vi "XY Fitting.vi"() -> ()   [LabVIEW 2020]
uses:
  <vilib>/Utility/miscctls.llb/LVAnnotationListTypeDef.ctl
  global/SettingVariable.vi
  <vilib>/Analysis/NI_AALPro.lvlib
panel:
  out "历史波形图":cluster{dbl, dbl, dbl[][]}(graph)
  out "左选标时刻":timestamp caption="左选标时刻：" format="%<%.2X %x>T"
  out "数据点数":i32 caption="数据点数："
  out "残差":dbl caption="残差："
  out "斜率":dbl caption="斜率："
  in  "在线数据":bool
  out "采样间隔":dbl
  out "开始时间":timestamp
  in  "x轴选择":u16(ring) caption="x轴选择："
  in  "y轴选择":u16(ring) caption="y轴选择："
  in  "打开文件":bool
  out "XY 图":cluster{dbl[], "Best Linear Fit":dbl[]}[](graph)
  out "提示信息":string="打开文件后，拖动波形图中的游标选取显示在XY图上的数据段，通过下拉框选择x和y轴对应的数据。"
  out "文件信息":string
  # "坐标轴与图例"
  # "拟合结果"
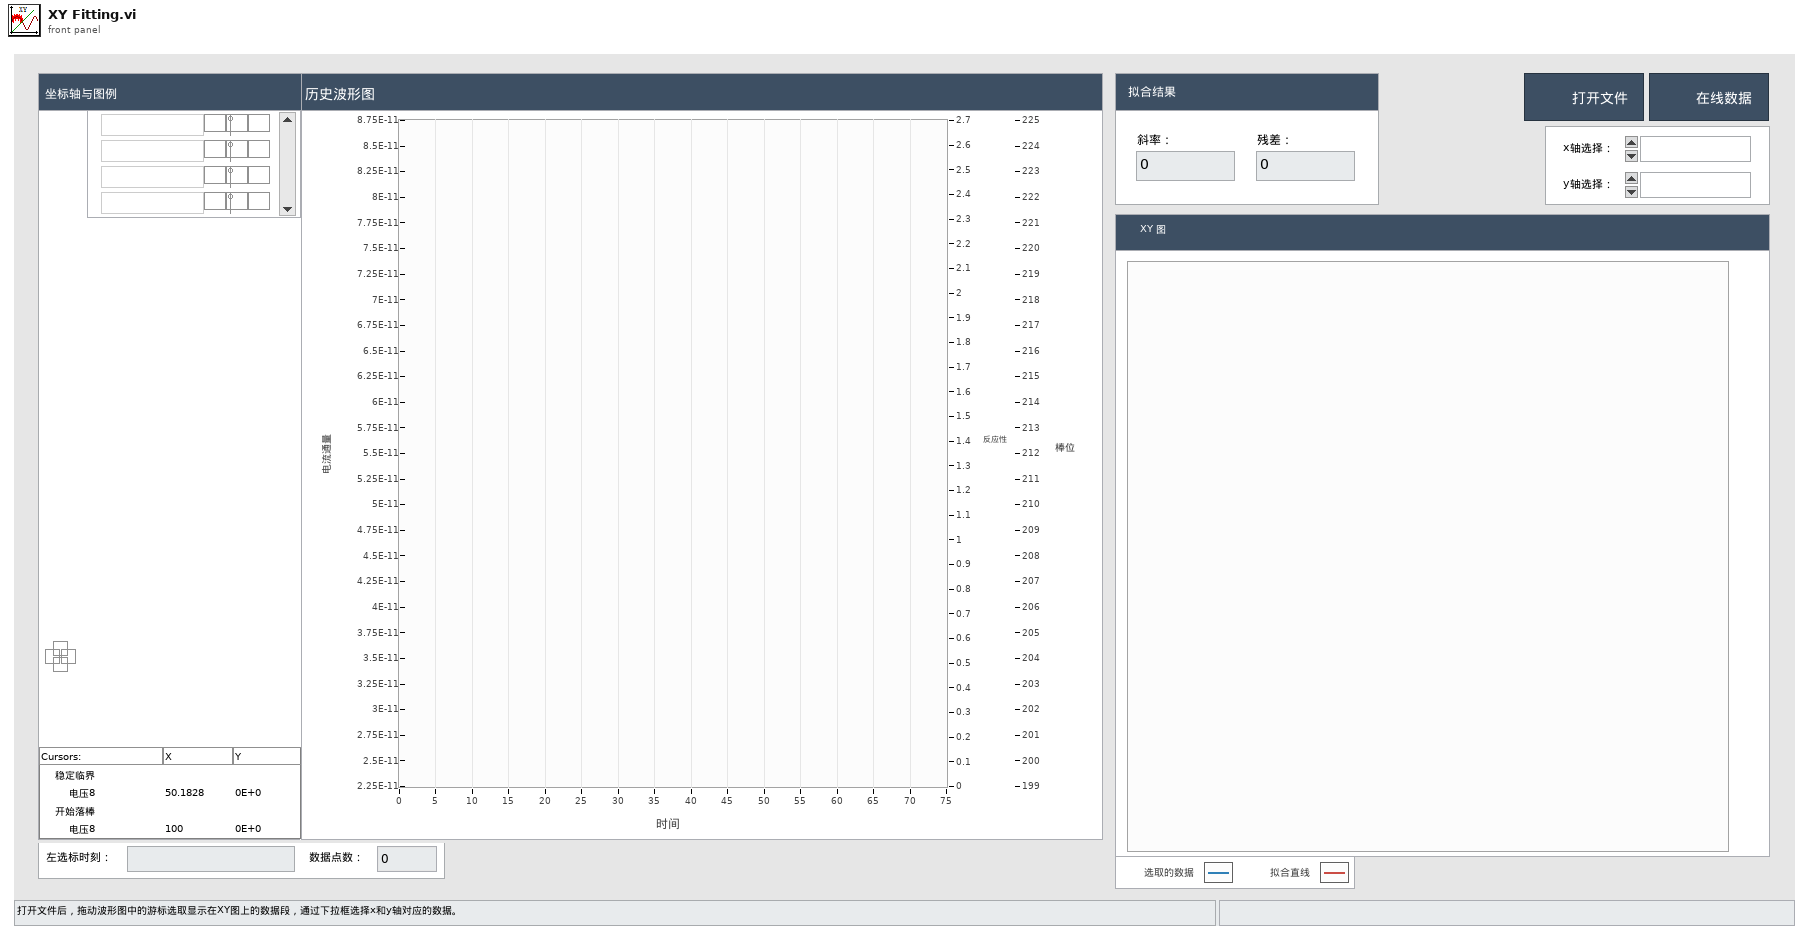
[diagram p1: front panel]
types:
  T1 = typedef "LVAnnotationListTypeDef.ctl" = cluster{"Name":string, "Color":u32, "Style":u8, "Point Style":u8, "Name Visible":bool, "Allow Drag":bool, "Annotation Mode":u32, "Plot":i32, "Index":i32, "Position":cluster{"X":dbl, "Y":dbl}, "X Scale":u32, "Y Scale":u32, "Show Arrow":bool, "Lock Name":bool, "Plot Area":i32, "Label Offset":cluster{"X":dbl, "Y":dbl}}[]
  T2 = cluster{"Name":string, "Color":u32, "Style":u8, "Point Style":u8, "Name Visible":bool, "Allow Drag":bool, "Annotation Mode":u32, "Plot":i32, "Index":i32, "Position":cluster{"X":dbl, "Y":dbl}, "X Scale":u32, "Y Scale":u32, "Show Arrow":bool, "Lock Name":bool, "Plot Area":i32, "Label Offset":cluster{"X":dbl, "Y":dbl}}
  T3 = typedef "LVCursorListTypeDef.ctl" = cluster{"Name":string, "Color":u32, "Style":u8, "Point Style":u8, "Name Visible":bool, "Allow Drag":bool, "Cursor Mode":u32, "Plot":i32, "Index":i32, "Position":cluster{"X":dbl, "Y":dbl}, "X Scale":u32, "Y Scale":u32, "Watch Plots":i32[], "Watch All Plots":bool, "Plot Area":i32, "Label Offset":cluster{"X":dbl, "Y":dbl}}[]
  T4 = cluster{"Name":string, "Color":u32, "Style":u8, "Point Style":u8, "Name Visible":bool, "Allow Drag":bool, "Cursor Mode":u32, "Plot":i32, "Index":i32, "Position":cluster{"X":dbl, "Y":dbl}, "X Scale":u32, "Y Scale":u32, "Watch Plots":i32[], "Watch All Plots":bool, "Plot Area":i32, "Label Offset":cluster{"X":dbl, "Y":dbl}}
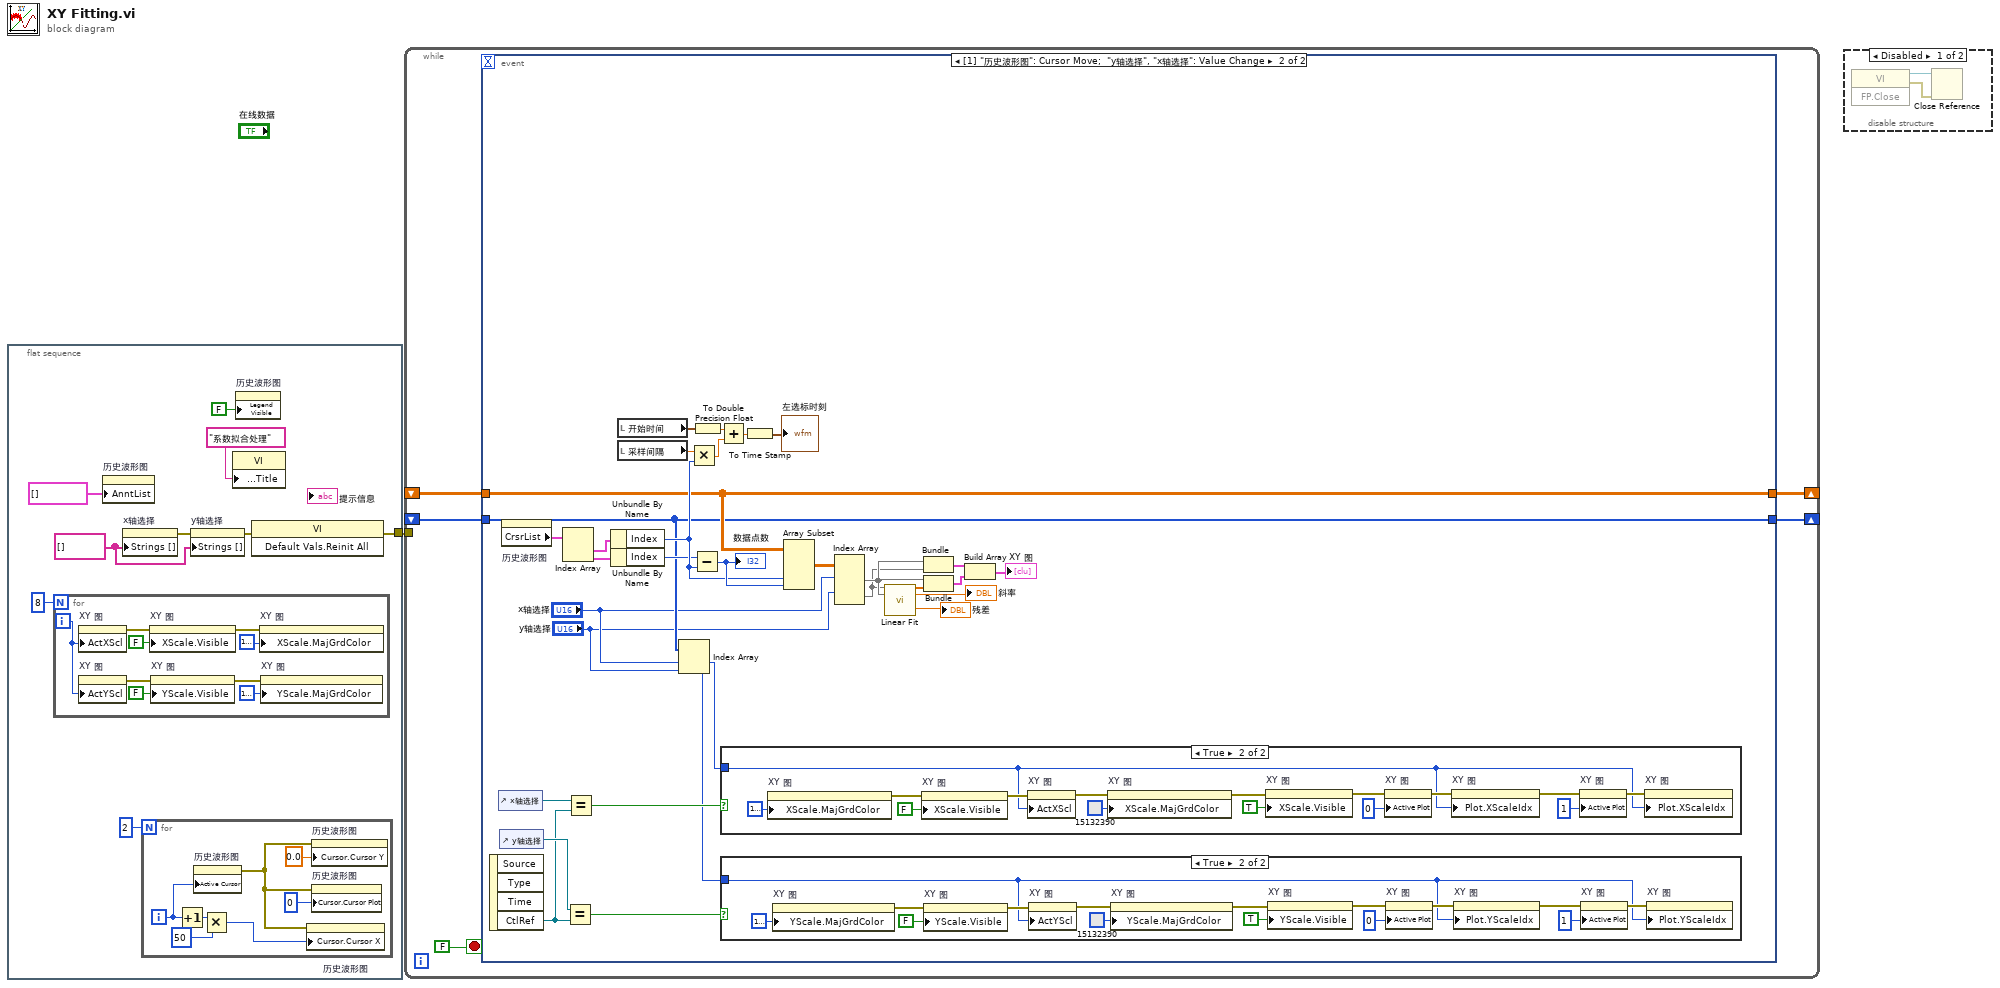
[diagram p0: block diagram]
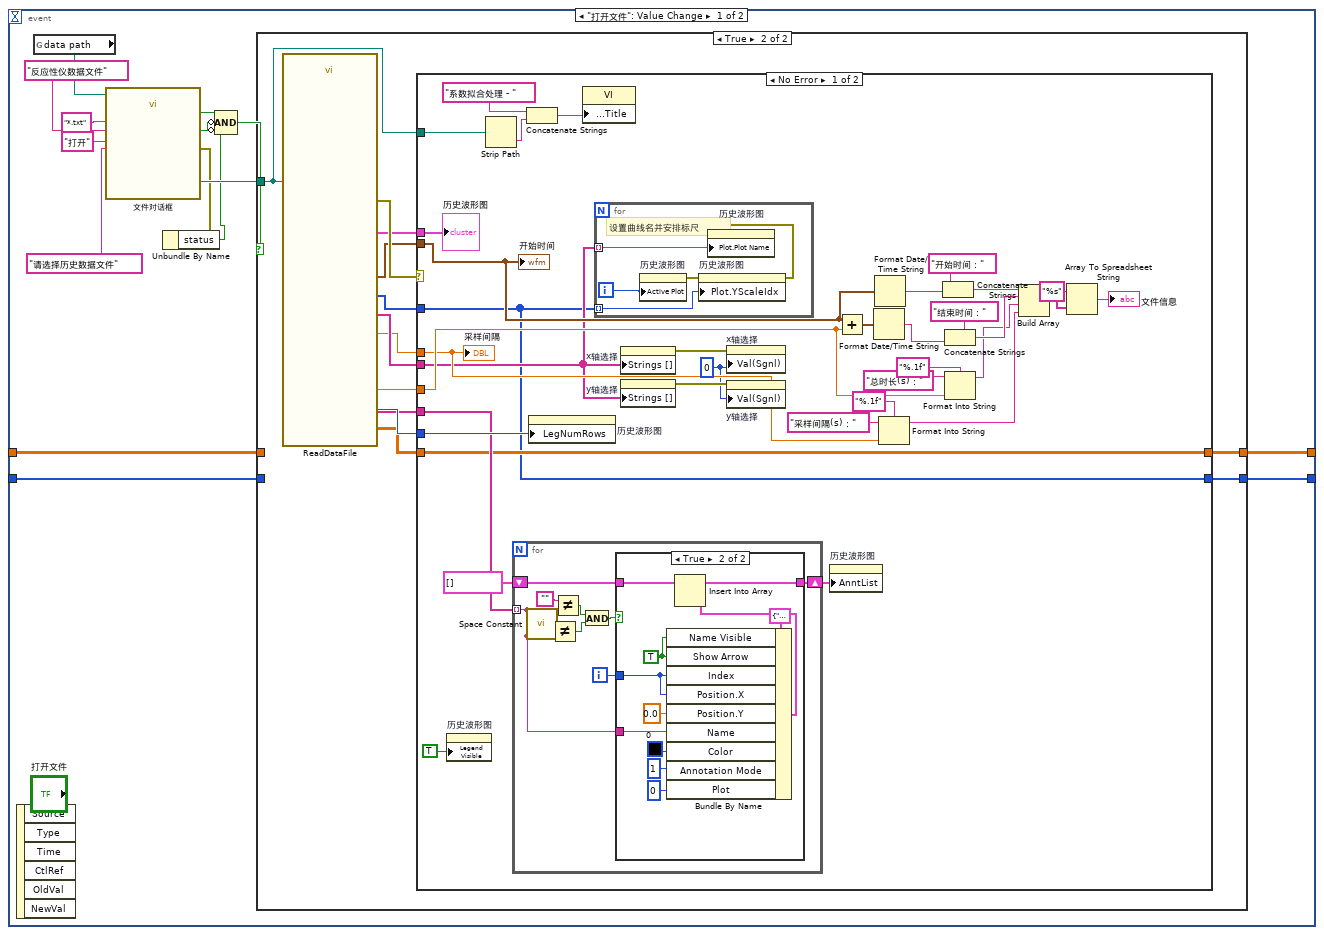
[diagram p2: hidden frame]
diagram:
  n1 = flat-sequence {
    tunnel: [w9] -> w1
    frame #0 {
      w3 = string[] [] ("Strings []")
      n2 = for {
        N: 8 -> [_]
        i -> [w11]
        n3 = property on="XY 图" class="XYGraph (strict)"("ActXScl"=w11) -> (error out=w18:errorcluster)  [unwired: 2 in, 1 out]
        n4 = property on="XY 图" class="XYGraph (strict)"("ActYScl"=w11) -> (error out=w13:errorcluster)  [unwired: 2 in, 1 out]
        n5 = property on="XY 图" class="XYGraph (strict)"(error in=w18, "XScale.Visible"=FALSE ("X Scale.Visible")) -> (error out=w17:errorcluster)  [unwired: 1 in, 1 out]
        n6 = property on="XY 图" class="XYGraph (strict)"(error in=w13, "YScale.Visible"=FALSE ("X Scale.Visible")) -> (error out=w14:errorcluster)  [unwired: 1 in, 1 out]
        n7 = property on="XY 图" class="XYGraph (strict)"(error in=w17, "XScale.MajGrdColor"=u32 16777216 ("X Scale.Grid Colors:Major Color")) -> ()  [unwired: 1 in, 2 out]
        n8 = property on="XY 图" class="XYGraph (strict)"(error in=w14, "YScale.MajGrdColor"=u32 16777216 ("X Scale.Grid Colors:Major Color")) -> ()  [unwired: 1 in, 2 out]
      }
      n9 = property on="历史波形图" class="WFGraph (strict)"("AnntList"=T1 [] ("Annotation List")) -> ()  [unwired: 2 in, 2 out]
      n10 = property on="x轴选择" class="Ring (strict)"("Strings []"=w3) -> (error out=w4:errorcluster)  [unwired: 2 in, 1 out]
      n11 = for {
        N: 2 -> [_]
        i -> [w24]
        n12 = Increment(x=w24) -> (x+1=w23:i32)
        n13 = property on="历史波形图" class="WFGraph (strict)"("Active Cursor"=w24) -> (error out=w20:errorcluster)  [unwired: 2 in, 1 out]
        n14 = Multiply(x=w23, y=50) -> (x*y=w21:i32)
        n15 = property on="历史波形图" class="WFGraph (strict)"(error in=w20, "Cursor.Cursor X"=w21) -> ()  [unwired: 1 in, 2 out]
        n16 = property on="历史波形图" class="WFGraph (strict)"(error in=w20, "Cursor.Cursor Y"=0.0 ("Cursor.Cursor Position:Cursor Y")) -> ()  [unwired: 1 in, 2 out]
        n17 = property on="历史波形图" class="WFGraph (strict)"(error in=w20, "Cursor.Cursor Plot"=0 ("Cursor.Cursor Index")) -> ()  [unwired: 1 in, 2 out]
      }
      n18 = property on="y轴选择" class="Ring (strict)"(error in=w4, "Strings []"=w3) -> (error out=w8:errorcluster)  [unwired: 1 in, 1 out]
      n19 = property class="VI"("Front Panel.Title"="系数拟合处理" ("Front Panel Window:Title")) -> ()  [unwired: 2 in, 2 out]
      n20 = property on="历史波形图" class="WFGraph (strict)"("Legend Visible"=FALSE ("Legend:Visible")) -> ()  [unwired: 2 in, 2 out]
      n21 = invoke class="VI" method="Default Vals.Reinit All"(error in=w8) -> (error out=w9:errorcluster)  [unwired: 2 in, 2 out]
    }
  }
  n22 = while {
    tunnel: w1 -> [_]
    shift-right: [w30] -> _
    shift-left: _ -> [w29]
    shift-right: [w28] -> _
    shift-left: _ -> [w27]
    stop <- FALSE stop-if-true
    n23 = event shown="[1] \"历史波形图\": Cursor Move;  \"y轴选择\", \"x轴选择\": Value Change" {
      selector: _ -> [_ _]
      dyn-events: _ -> [_ _]
      timeout: _ -> [_ _]
      tunnel: [w35 w131] -> w30
      tunnel: w29 -> [w34 w131]
      tunnel: [w33 w130] -> w28
      tunnel: w27 -> [w32 w130]
      event "打开文件": Value Change {
        n24 = event-data() -> ()  [unwired: 1 in, 6 out]
        n25 = global read "SettingVariable.vi" "data path"() -> (w36:path)
        n26 = call "文件对话框"("start path"=w36, "prompt"="请选择历史数据文件", "button label"="打开", "pattern (all files)"="*.txt", "pattern label"="反应性仪数据文件") -> ("selected path"=w46:path, "exists"=w40:bool, "cancelled"=w39:bool, "error out"=w41:errorcluster)  [unwired: 7 in]
        n27 = Unbundle By Name(w41) -> ("status"=w38:bool)
        n28 = Compound Arithmetic op=AND(w40, invert w39, invert w38) -> (w37:bool)
        n29 = case shown="True" w37 {
          tunnel: w46 -> [_ w52]
          tunnel: [w48 w50] -> w35
          tunnel: w34 -> [w48 _]
          tunnel: [w47 w49] -> w33
          tunnel: w32 -> [w47 _]
          frame False {
          }
          frame True {
            n30 = call "ReadDataFile.vi"("file path"=w52) -> ("曲线对应标尺编号"=w56:i32[], "全部数据"=w51:dbl[][], "曲线名"=w55:string[], "时间间隔"=w54:dbl, "曲线数"=w58:i32, "开始时间"=w53:timestamp, "总时长(s)"=w59:dbl, "error out"=w61:errorcluster, "备注数组"=w57:string[], "波形簇"=w60:cluster{dbl, dbl, dbl[][]})  [unwired: 2 in, 3 out]
            n31 = case shown="No Error" w61 {
              tunnel: w60 -> [w96 _]
              tunnel: w59 -> [w86 _]
              tunnel: w58 -> [w95 _]
              tunnel: w57 -> [w92 _]
              tunnel: w56 -> [w65 w123]
              tunnel: w55 -> [w66 _]
              tunnel: w54 -> [w68 _]
              tunnel: w53 -> [w69 _]
              tunnel: w52 -> [w71 _]
              tunnel: w51 -> [w67 w124]
              tunnel: [w67 w124] -> w50
              tunnel: [w65 w123] -> w49
              frame No Error {
                w62 = u16 0 ("Value (Signaling)")
                n32 = property on="历史波形图" class="WFGraph (strict)"("Legend Visible"=TRUE ("Legend:Visible")) -> ()  [unwired: 2 in, 2 out]
                n33 = Strip Path(path=w71) -> (name=w72:string)  [unwired: 1 out]
                n34 = for {
                  tunnel: w92 -> [w105] mode=indexing
                  shift-right: [w107] -> w94
                  shift-left: T1 [] ("注释列表") -> [w108]
                  i -> [w109]
                  n35 = call <vilib>:"Space Constant.vi"() -> ("String"=w110:string)
                  n36 = Not Equal?(x=w110, y=w105) -> (x != y?=w103:bool)
                  n37 = Not Equal?(x="", y=w105) -> (x != y?=w104:bool)
                  n38 = And(x=w104, y=w103) -> (x .and. y?=w102:bool)
                  n39 = case shown="True" w102 {
                    tunnel: w105 -> [_ w118]
                    tunnel: w109 -> [_ w112]
                    tunnel: w108 -> [w111 w122]
                    tunnel: [w111 w121] -> w107
                    frame False {
                    }
                    frame True {
                      w120 = TRUE ("Show Arrow")
                      n40 = Bundle By Name(cluster=T2 {"Name"="", "Color"=0, "Style"=0, "Point Style"=0, "Name Visible"=FALSE, "Allow Drag"=FALSE, "Annotation Mode"=0, "Plot"=0, "Index"=0, "Position"={"X"=0.0, "Y"=0.0}, "X Scale"=0, "Y Scale"=0, "Show Arrow"=FALSE, "Lock Name"=FALSE, "Plot Area"=0, "Label Offset"={"X"=0.0, "Y"=0.0}} ("元素"), "Name Visible"=w120, "Show Arrow"=w120, "Index"=w112, "Position.X"=w112, "Position.Y"=0.0 ("Y"), "Name"=w118, "Color"=u32 0, "Annotation Mode"=u32 1, "Plot"=0) -> (w119:T2)
                      n41 = Insert Into Array(array=w122, new element=w119) -> (w121:T1)  [unwired: 1 in]
                    }
                  }
                }
                n42 = Concatenate Strings("系数拟合处理 - " ("string"), w72) -> (w73:string)
                n43 = property on="历史波形图" class="WFGraph (strict)"("LegNumRows"=w95) -> ()  [unwired: 2 in, 2 out]
                n44 = property class="VI"("Front Panel.Title"=w73) -> ()  [unwired: 2 in, 2 out]
                n45 = for {
                  tunnel: w65 -> [w99] mode=indexing
                  tunnel: w66 -> [w97] mode=indexing
                  i -> [w98]
                  # "设置曲线名并安排标尺"
                  n46 = property on="历史波形图" class="WFGraph (strict)"("Active Plot"=w98) -> (error out=w101:errorcluster)  [unwired: 2 in, 1 out]
                  n47 = property on="历史波形图" class="WFGraph (strict)"(error in=w101, "Plot.YScaleIdx"=w99) -> (error out=w100:errorcluster)  [unwired: 1 in, 1 out]
                  n48 = property on="历史波形图" class="WFGraph (strict)"(error in=w100, "Plot.Plot Name"=w97) -> ()  [unwired: 1 in, 2 out]
                }
                n49 = property on="x轴选择" class="Ring (strict)"("Strings []"=w66) -> (error out=w64:errorcluster)  [unwired: 2 in, 1 out]
                n50 = property on="y轴选择" class="Ring (strict)"("Strings []"=w66) -> (error out=w63:errorcluster)  [unwired: 2 in, 1 out]
                n51 = property on="x轴选择" class="Ring (strict)"(error in=w64, "Val(Sgnl)"=w62) -> ()  [unwired: 1 in, 2 out]
                n52 = property on="y轴选择" class="Ring (strict)"(error in=w63, "Val(Sgnl)"=w62) -> ()  [unwired: 1 in, 2 out]
                n53 = property on="历史波形图" class="WFGraph (strict)"("AnntList"=w94) -> ()  [unwired: 2 in, 2 out]
                n54 = Add(x=w69, y=w86) -> (x+y=w91:timestamp)
                n55 = Format Date/Time String(seconds (now)=w91) -> (date/time string=w87:string)  [unwired: 2 in]
                n56 = Format Date/Time String(seconds (now)=w69) -> (date/time string=w89:string)  [unwired: 2 in]
                n57 = Format Into String(format string="%.1f", initial string="采样间隔(s)：", w68) -> (resulting string=w78:string)  [unwired: 1 in, 1 out]
                n58 = Concatenate Strings("开始时间：" ("string"), w89) -> (w83:string)
                n59 = Concatenate Strings("结束时间：" ("string"), w87) -> (w80:string)
                n60 = Format Into String(format string="%.1f", initial string="总时长(s)：", w86) -> (resulting string=w79:string)  [unwired: 1 in, 1 out]
                n61 = Build Array(w83, w80, w79, w78) -> (w82:string[])
                n62 = Array To Spreadsheet String(array=w82, 3:"%s" ("format string")) -> (spreadsheet string=→"文件信息":string)  [unwired: 1 in]
                "历史波形图" <- w96
                "开始时间" <- w69
                "采样间隔" <- w68
              }
              frame Error {
              }
            }
          }
        }
      }
      event "历史波形图": Cursor Move; "y轴选择", "x轴选择": Value Change {
        n63 = event-data() -> ("CtlRef"=w133:refnum<vi>)  [unwired: 1 in, 3 out]
        n64 = control-ref of="x轴选择"() -> (w134:refnum<vi>)
        n65 = control-ref of="y轴选择"() -> (w144:refnum<vi>)
        n66 = property on="历史波形图" class="WFGraph (strict)"() -> ("CrsrList"=w154:T3)  [unwired: 2 in, 2 out]
        n67 = Index Array(array=w154) -> (element #1=w155:T4, element #2=w156:T4)  [unwired: 2 in]
        n68 = Equal?(x=w144, y=w133) -> (x = y?=w143:bool)
        n69 = Equal?(x=w134, y=w133) -> (x = y?=w132:bool)
        n70 = Unbundle By Name(w155) -> ("Index"=w148:i32)
        n71 = Unbundle By Name(w156) -> ("Index"=w147:i32)
        n72 = local read "开始时间"() -> (w146:timestamp)
        n73 = local read "采样间隔"() -> (w145:dbl)
        n74 = Index Array(array=w130, index #1="x轴选择", index #2="y轴选择") -> (element #1=w127:i32, element #2=w126:i32)
        n75 = Multiply(x=w145, y=w148) -> (x*y=w149:dbl)
        n76 = Subtract(x=w147, y=w148) -> (x-y=w153:i32)
        "数据点数" <- w153
        n77 = To Double Precision Float(number=w146) -> (double precision float=w152:dbl)
        n78 = Add(x=w152, y=w149) -> (x+y=w151:dbl)
        n79 = case shown="True" w132 {
          tunnel: w127 -> [_ w162]
          frame False {
          }
          frame True {
            n80 = property on="XY 图" class="XYGraph (strict)"("XScale.MajGrdColor"=u32 16777216 ("X Scale.Grid Colors:Major Color")) -> (error out=w158:errorcluster)  [unwired: 2 in, 1 out]
            n81 = property on="XY 图" class="XYGraph (strict)"(error in=w158, "XScale.Visible"=FALSE ("X Scale.Visible")) -> (error out=w167:errorcluster)  [unwired: 1 in, 1 out]
            n82 = property on="XY 图" class="XYGraph (strict)"(error in=w167, "ActXScl"=w162) -> (error out=w160:errorcluster)  [unwired: 1 in, 1 out]
            n83 = property on="XY 图" class="XYGraph (strict)"(error in=w160, "XScale.MajGrdColor"=u32 15132390 ("X Scale.Grid Colors:Major Color")) -> (error out=w159:errorcluster)  [unwired: 1 in, 1 out]
            n84 = property on="XY 图" class="XYGraph (strict)"(error in=w159, "XScale.Visible"=TRUE ("X Scale.Visible")) -> (error out=w168:errorcluster)  [unwired: 1 in, 1 out]
            n85 = property on="XY 图" class="XYGraph (strict)"(error in=w168, "Active Plot"=0 ("Active X Scale")) -> (error out=w169:errorcluster)  [unwired: 1 in, 1 out]
            n86 = property on="XY 图" class="XYGraph (strict)"(error in=w169, "Plot.XScaleIdx"=w162) -> (error out=w171:errorcluster)  [unwired: 1 in, 1 out]
            n87 = property on="XY 图" class="XYGraph (strict)"(error in=w171, "Active Plot"=1 ("Active X Scale")) -> (error out=w170:errorcluster)  [unwired: 1 in, 1 out]
            n88 = property on="XY 图" class="XYGraph (strict)"(error in=w170, "Plot.XScaleIdx"=w162) -> ()  [unwired: 1 in, 2 out]
          }
        }
        n89 = case shown="True" w143 {
          tunnel: w126 -> [_ w177]
          frame False {
          }
          frame True {
            n90 = property on="XY 图" class="XYGraph (strict)"("YScale.MajGrdColor"=u32 16777216 ("X Scale.Grid Colors:Major Color")) -> (error out=w173:errorcluster)  [unwired: 2 in, 1 out]
            n91 = property on="XY 图" class="XYGraph (strict)"(error in=w173, "YScale.Visible"=FALSE ("X Scale.Visible")) -> (error out=w182:errorcluster)  [unwired: 1 in, 1 out]
            n92 = property on="XY 图" class="XYGraph (strict)"(error in=w182, "ActYScl"=w177) -> (error out=w176:errorcluster)  [unwired: 1 in, 1 out]
            n93 = property on="XY 图" class="XYGraph (strict)"(error in=w176, "YScale.MajGrdColor"=u32 15132390 ("X Scale.Grid Colors:Major Color")) -> (error out=w175:errorcluster)  [unwired: 1 in, 1 out]
            n94 = property on="XY 图" class="XYGraph (strict)"(error in=w175, "YScale.Visible"=TRUE ("X Scale.Visible")) -> (error out=w181:errorcluster)  [unwired: 1 in, 1 out]
            n95 = property on="XY 图" class="XYGraph (strict)"(error in=w181, "Active Plot"=0 ("Active X Scale")) -> (error out=w180:errorcluster)  [unwired: 1 in, 1 out]
            n96 = property on="XY 图" class="XYGraph (strict)"(error in=w180, "Plot.YScaleIdx"=w177) -> (error out=w178:errorcluster)  [unwired: 1 in, 1 out]
            n97 = property on="XY 图" class="XYGraph (strict)"(error in=w178, "Active Plot"=1 ("Active X Scale")) -> (error out=w179:errorcluster)  [unwired: 1 in, 1 out]
            n98 = property on="XY 图" class="XYGraph (strict)"(error in=w179, "Plot.YScaleIdx"=w177) -> ()  [unwired: 1 in, 2 out]
          }
        }
        n99 = To Time Stamp(1:w151) -> (0:→"左选标时刻":timestamp)
        n100 = Array Subset(array=w131, index (col)=w148, length (col)=w153) -> (w142:dbl[][])  [unwired: 2 in]
        n101 = Index Array(array=w142, index (row) #1="x轴选择", index (row) #2="y轴选择") -> (element #1=w140:dbl[], element #2=w139:dbl[])  [unwired: 2 in]
        n102 = call <vilib>:"Linear Fit.vi"("Y"=w139, "X"=w140) -> ("Best Linear Fit"=w141:dbl[], "slope"=→"斜率":dbl, "residue"=→"残差":dbl)  [unwired: 9 in, 2 out]
        n103 = Bundle(w140, w139) -> (w138:cluster{dbl[], dbl[]})  [unwired: 1 in]
        n104 = Bundle(w140, "Best Linear Fit"=w141) -> (w137:cluster{dbl[], "Best Linear Fit":dbl[]})  [unwired: 1 in]
        n105 = Build Array(w138, w137) -> (→"XY 图":cluster{dbl[], "Best Linear Fit":dbl[]}[])
      }
    }
  }
  n106 = disable-structure shown="Disabled" {
    frame Disabled {
      n107 = invoke class="VI" method="FP.Close"() -> (reference out=w188:refnum<vi>, error out=w187:errorcluster)  [unwired: 3 in, 1 out]
      n108 = Close Reference(reference=w188, error in (no error)=w187) -> ()  [unwired: 1 out]
    }
    frame Enabled {
    }
  }
